vi "RunLogRecord.vi"(8 "error in (no error)":errorcluster, 11 "Config":T1={"LogName"="", "Level"=enum."Info", "LogFolder"=path "", "MaxFileSize"=0, "FileExtension"="", "TimeSytle"="", "LogStyle"=""}) -> (0 "error out":errorcluster)   [LabVIEW 2016, in "Log4Lv.lvlib"]
doc: "Use this template to build a VI to use as a subVI."
uses:
  Log4Lv.lvlib
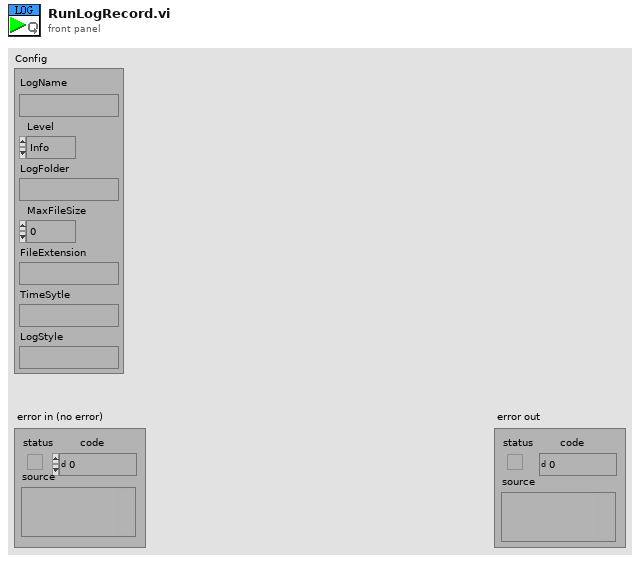
[diagram p1: front panel]
types:
  T1 = cluster{"LogName":string, "Level":enum16{"Disable", "Error", "Warn", "Info", "Debug"}, "LogFolder":path, "MaxFileSize":i32, "FileExtension":string, "TimeSytle":string, "LogStyle":string}
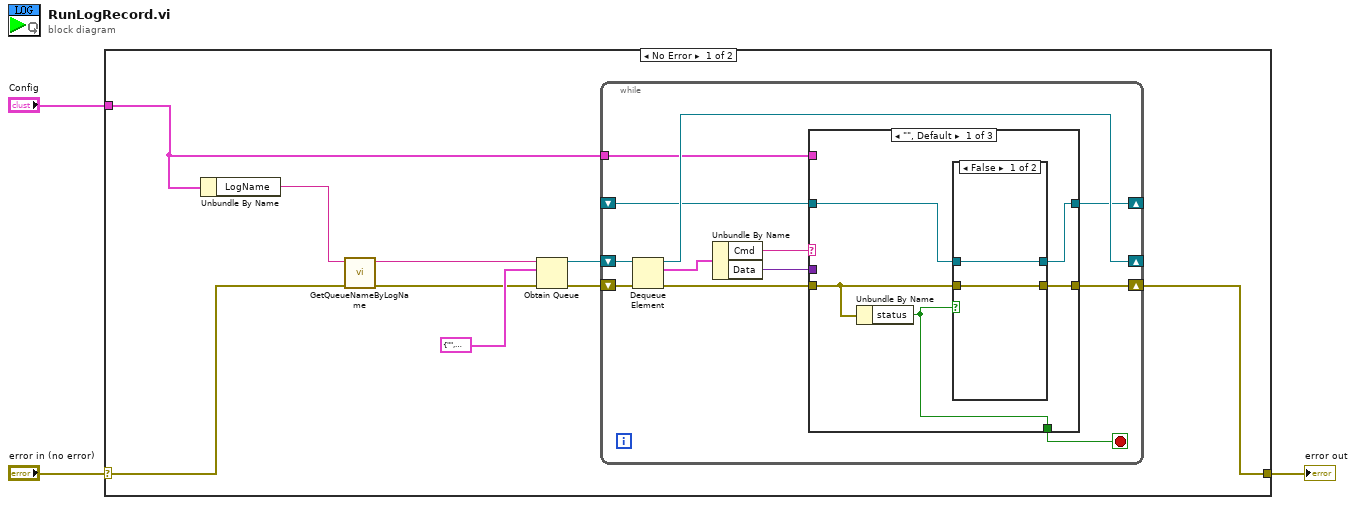
[diagram p0: block diagram]
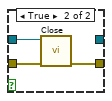
[diagram p2: hidden frame]
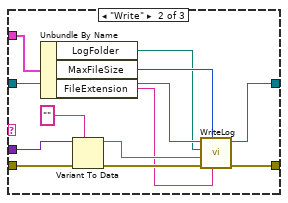
[diagram p3: hidden frame]
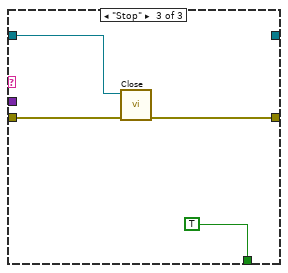
[diagram p4: hidden frame]
diagram:
  n1 = case shown="No Error" "error in (no error)" {
    selector: "error in (no error)" -> [w8 w51]
    tunnel: [w4 w51] -> w2
    tunnel: "Config" -> [w9 _]
    frame No Error {
      n2 = Unbundle By Name(w9) -> ("LogName"=w6:string)
      n3 = call "GetQueueNameByLogName.vi"("error in (no error)"=w8, "LogName"=w6) -> ("error out"=w7:errorcluster, "QueueName"=w5:string)  [unwired: 8 in]
      n4 = Obtain Queue(name (unnamed)=w5, element data type=cluster{"Cmd":string, "Data":variant} {"Cmd"="", "Data"=variant}, error in (no error)=w7) -> (queue out=w11:refnum<queue>, error out=w10:errorcluster)  [unwired: 2 in, 1 out]
      n5 = while {
        shift-right: [w18] -> w4
        shift-left: w10 -> [w23]
        shift-right: [w16] -> _
        shift-left: w11 -> [w24]
        tunnel: w9 -> [w15]
        shift-right: [w13] -> _
        shift-left: _ -> [w14]
        stop <- w17 stop-if-true
        n6 = Dequeue Element(queue=w24, error in (no error)=w23) -> (queue out=w16:refnum<queue>, element=w22:cluster{"Cmd":string, "Data":variant}, error out=w21:errorcluster)  [unwired: 1 in, 1 out]
        n7 = Unbundle By Name(w22) -> ("Cmd"=w20:string, "Data"=w19:variant)
        n8 = case shown="\"\", Default" w20 {
          tunnel: w21 -> [w29 w46 w49]
          tunnel: w19 -> [_ w45 _]
          tunnel: [w28 w41 w48] -> w18
          tunnel: [w27 _ TRUE] -> w17
          tunnel: w15 -> [_ w43 _]
          tunnel: w14 -> [w26 w39 w47]
          tunnel: [w25 w38 _] -> w13
          frame "", Default {
            n9 = Unbundle By Name(w29) -> ("status"=w27:bool)
            n10 = case shown="False" w27 {
              tunnel: w29 -> [w31 w34]
              tunnel: [w31 w33] -> w28
              tunnel: w26 -> [w30 w32]
              tunnel: [w30 _] -> w25
              frame False {
              }
              frame True {
                n11 = call "Close.vi"("error in (no error)"=w34, "Logfile Ref In"=w32) -> ("error out"=w33:errorcluster)  [unwired: 9 in]
              }
            }
          }
          frame "Write" {
            n12 = Unbundle By Name(w43) -> ("LogFolder"=w36:path, "MaxFileSize"=w37:i32, "FileExtension"=w35:string)
            n13 = Variant To Data(error in=w46, type="", Variant=w45) -> (data=w40:string, error out=w42:errorcluster)
            n14 = call "WriteLog.vi"("FileExtension"=w35, "MaxFileSize"=w37, "error in (no error)"=w42, "Log"=w40, "LogFolder"=w36, "LogfileRef In"=w39) -> ("error out"=w41:errorcluster, "LogfileRef Out"=w38:refnum<file>)  [unwired: 4 in]
          }
          frame "Stop" {
            n15 = call "Close.vi"("error in (no error)"=w49, "Logfile Ref In"=w47) -> ("error out"=w48:errorcluster)  [unwired: 9 in]
          }
        }
      }
    }
    frame Error {
    }
  }
  "error out" <- w2
